vi "10SOCdischarge.vi"(0 "Battery Detect Voltage (0V)":dbl format="%#.6g", 1 "VISA resource name":refnum<visa-resource-name>, 2 "Path":path, 3 "DAQmx Task Name":refnum<k21>, 5 "Voltage Setpoint (0 V)":dbl format="%#.6g", 7 "Current Setpoint (0 A)":dbl format="%#.6g", 9 "Power Setpoint (0 W)":dbl format="%#.6g", 11 "Resistance Setpoint (0 Ohms)":dbl format="%#.6g", 12 "Discharge time":dbl, 13 "Task error in":errorcluster, 14 "error in (no error)":errorcluster) -> (4 "VISA resource name out":refnum<visa-resource-name>, 6 "Filename Out":path, 8 "task out":refnum<k21>, 10 "Task error out 2":errorcluster, 15 "error out":errorcluster)   [LabVIEW 2020]
uses:
  <vilib>/DAQmx/read.llb/DAQmx Read (Analog 1D DBL NChan 1Samp).vi
  <vilib>/DAQmx/miscellaneous.llb/DAQmx Fill In Error Info.vi
  <instrlib>/NH Research Regenerative Test Series/Public/Data/Read (Ave Current).vi
  <instrlib>/NH Research Regenerative Test Series/Public/Data/Low Level/Fetch (Ave Voltage).vi
  <instrlib>/NH Research Regenerative Test Series/Public/Data/Low Level/Fetch (Ave True Power).vi
  <instrlib>/NH Research Regenerative Test Series/NH Research Regenerative Test Series.lvlib
panel:
  out "Ave Current (A)":dbl
  out "Ave Voltage (V)":dbl
  out "Ave True Power (W)":dbl
  out "Status Byte Register":T1
  in  "Logical Instrument Number":u32=1
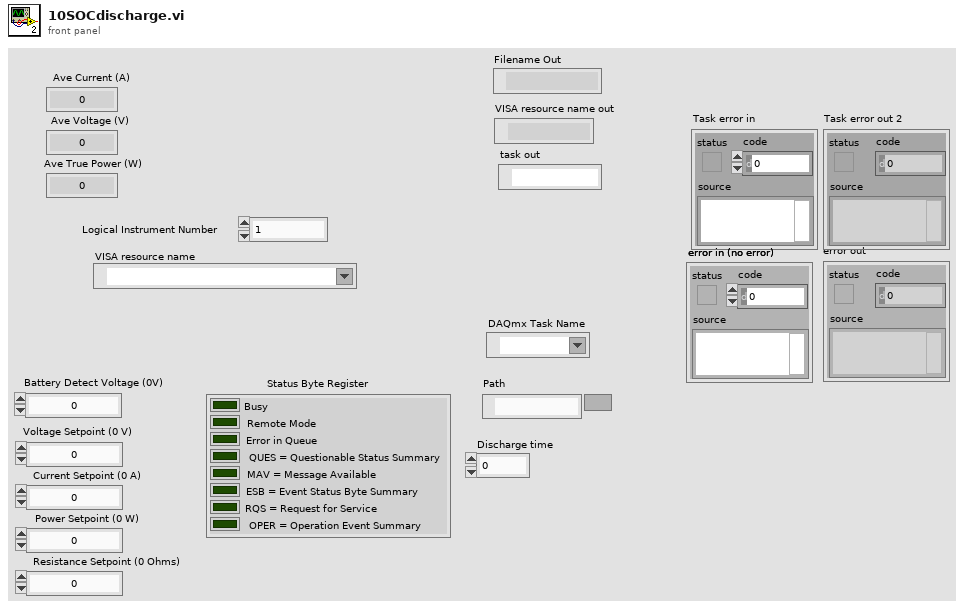
[diagram p1: front panel]
types:
  T1 = cluster{"Busy":bool, "Remote Mode":bool, "Error in Queue":bool, "QUES = Questionable Status Summary":bool, "MAV = Message Available":bool, "ESB = Event Status Byte Summary":bool, "RQS = Request for Service":bool, "OPER = Operation Event Summary":bool}
  T2 = cluster{"data[0]":dbl, "data[1]":dbl, "data[2]":dbl, "data[3]":dbl, "data[4]":dbl, "data[5]":dbl, "data[6]":dbl, "data[7]":dbl, "data[8]":dbl}
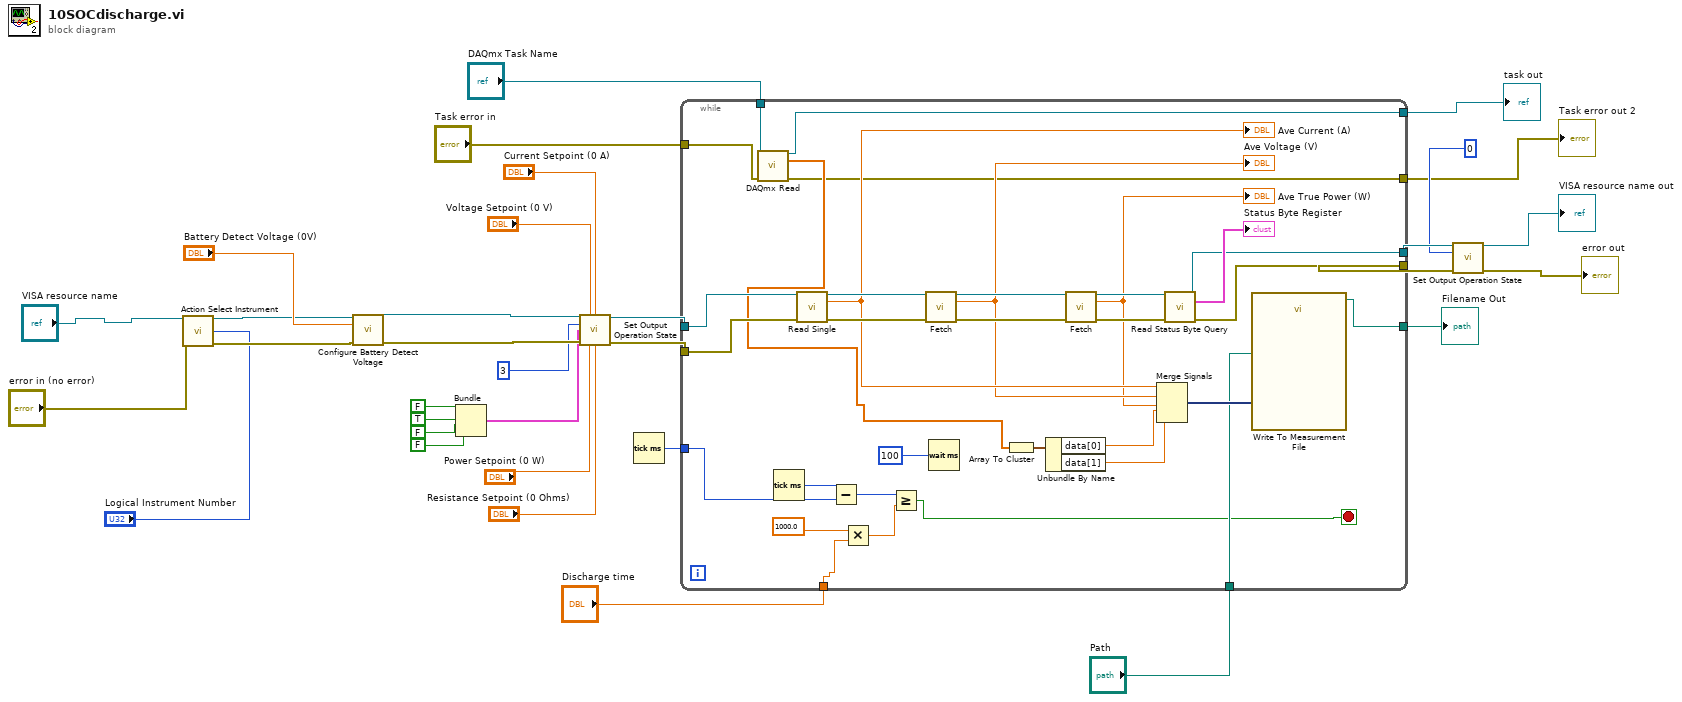
[diagram p0: block diagram]
diagram:
  n1 = call <instrlib>:"Action Select Instrument.vi"("VISA resource name"="VISA resource name", "Logical Instrument Number"="Logical Instrument Number", "error in (no error)"="error in (no error)") -> ("VISA resource name out"=w28:refnum<visa-resource-name>, "error out"=w27:errorcluster)  [unwired: 11 in]
  n2 = call <vilib>:"Configure Battery Detect Voltage.vi"("VISA resource name"=w28, "Battery Detect Voltage (0V)"="Battery Detect Voltage (0V)", "error in (no error)"=w27) -> ("VISA resource name out"=w26:refnum<visa-resource-name>, "error out"=w25:errorcluster)  [unwired: 11 in]
  n3 = Bundle(FALSE, TRUE, FALSE, FALSE) -> (w12:cluster{bool, bool, bool, bool})  [unwired: 1 in]
  n4 = call <vilib>:"Set Output Operation State.vi"("VISA resource name"=w26, "Voltage Setpoint (0 V)"="Voltage Setpoint (0 V)", "Current Setpoint (0 A)"="Current Setpoint (0 A)", "Mode (0: Off)"=3, "Enable"=w12, "error in (no error)"=w25, "Power Setpoint (0 W)"="Power Setpoint (0 W)", "Resistance Setpoint (0 Ohms)"="Resistance Setpoint (0 Ohms)") -> ("VISA resource name out"=w21:refnum<visa-resource-name>, "error out"=w20:errorcluster)  [unwired: 6 in]
  n5 = Tick Count (ms)() -> (millisecond timer value=w8:u32)
  n6 = while {
    tunnel: w21 -> [w59]
    tunnel: w20 -> [w58]
    tunnel: [w56] -> w24
    tunnel: [w55] -> w23
    tunnel: "Discharge time" -> [w39]
    tunnel: "Path" -> [w50]
    tunnel: "DAQmx Task Name" -> [w49]
    tunnel: w8 -> [w38]
    tunnel: [w37] -> w7
    tunnel: [w36] -> w4
    tunnel: [w35] -> w3
    tunnel: "Task error in" -> [w34]
    stop <- w40 stop-if-true
    n7 = call-poly <vilib>:"DAQmx Read.vi"("task/channels in"=w49, "error in"=w34) -> ("task out"=w36:refnum<k21>, "data"=w48:dbl[], "error out"=w35:errorcluster)  [unwired: 11 in]
    n8 = Tick Count (ms)() -> (millisecond timer value=w44:u32)
    n9 = call-poly <instrlib>:"Read Single.vi"("VISA resource name"=w59, "error in (no error)"=w58) -> ("VISA resource name out"=w64:refnum<visa-resource-name>, "Ave Current (A)"=w54:dbl, "error out"=w65:errorcluster)  [unwired: 11 in]
    "Ave Current (A)" <- w54
    n10 = Subtract(x=w44, y=w38) -> (x-y=w43:u32)
    n11 = Multiply(x=1000.0, y=w39) -> (x*y=w41:dbl)
    n12 = Greater Or Equal?(x=w43, y=w41) -> (x >= y?=w40:bool)
    n13 = call-poly <instrlib>:"Fetch.vi"("VISA resource name"=w64, "error in (no error)"=w65) -> ("VISA resource name out"=w63:refnum<visa-resource-name>, "Ave Voltage (V)"=w53:dbl, "error out"=w62:errorcluster)  [unwired: 11 in]
    "Ave Voltage (V)" <- w53
    n14 = Wait (ms)(milliseconds to wait=100) -> ()  [unwired: 1 out]
    n15 = Array To Cluster(array=w48) -> (cluster=w47:T2)
    n16 = Unbundle By Name(w47) -> ("data[0]"=w46:dbl, "data[1]"=w45:dbl)
    n17 = call-poly <instrlib>:"Fetch.vi"("VISA resource name"=w63, "error in (no error)"=w62) -> ("VISA resource name out"=w61:refnum<visa-resource-name>, "Ave True Power (W)"=w52:dbl, "error out"=w60:errorcluster)  [unwired: 11 in]
    "Ave True Power (W)" <- w52
    n18 = Merge Signals "Merge Signals"(w54, w53, w52, w46, w45) -> (w66:dynamicdata)
    n19 = call <instrlib>:"Read Status Byte Query.vi"("VISA resource name"=w61, "error in (no error)"=w60) -> ("VISA resource name out"=w56:refnum<visa-resource-name>, "Status Byte Register"=→"Status Byte Register":T1, "error out"=w55:errorcluster)  [unwired: 11 in]
    n20 = call "Write To Measurement File"("Signals"=w66, "Filename"=w50) -> ("Filename Out"=w37:path)  [unwired: 15 in, 2 out]
  }
  "Filename Out" <- w7
  "task out" <- w4
  "Task error out 2" <- w3
  n21 = call <vilib>:"Set Output Operation State.vi"("VISA resource name"=w24, "Mode (0: Off)"=0, "error in (no error)"=w23) -> ("VISA resource name out"=→"VISA resource name out":refnum<visa-resource-name>, "error out"=→"error out":errorcluster)  [unwired: 11 in]
